vi "MaxiGauge EPICS.vi"() -> ()   [LabVIEW 2015]
uses:
  <vilib>/Platform/TimedLoop/XDataNode/timing_clust.ctl
  <vilib>/Platform/TimedLoop/XDataNode/nitl_modes.ctl
  <vilib>/Platform/TimedLoop/XDataNode/wakeup.ctl
  <userlib>/caLab/Private/Get_PV-1D.vi
  <userlib>/caLab/Private/Put_DBL-1D_PV-1D.vi
  <vilib>/platform/TimedLoop/XDataNode/XDataNode.xnode
  <vilib>/Platform/TimedLoop/XDataNode/XDNodeRunTimeDep.lvlib
panel:
  out "Finished Late? [i-1]":bool
  out "Actual Start [i]":i64
  out "Relay E":string
  out "Error out":errorcluster
  out "Maxigauge COMPORT":string
  out "APX:SEN6_STS":bool
  out "APX:SEN5_STS":bool
  out "APX:SEN4_STS":bool
  out "APX:SEN3_STS":bool
  out "APX:SEN2_STS":bool
  out "APX:SEN1_STS":bool
  out "APX:SEN6_VAL":dbl
  out "APX:SEN5_VAL":dbl
  out "APX:SEN4_VAL":dbl format="%#_3g"
  out "APX:SEN3_VAL":dbl format="%#_3g"
  out "APX:SEN2_VAL":dbl format="%#_3g"
  out "APX:SEN1_VAL":dbl
  out "APX:SEN6_OFF":bool
  out "APX:SEN6_ON":bool
  out "APX:SEN5_OFF":bool
  out "APX:SEN5_ON":bool
  out "APX:SEN4_OFF":bool
  out "APX:SEN4_ON":bool
  out "APX:SEN3_OFF":bool
  out "APX:SEN3_ON":bool
  out "APX:SEN2_OFF":bool
  out "APX:SEN2_ON":bool
  out "APX:SEN1_OFF":bool
  out "APX:SEN1_ON":bool
  out "APX:SP_SES100":bool
  out "MaxiGauge":dbl[](array[numeric])
  out "P torr":dbl[](array[numeric])
  in  "STOP":bool
  # "Ch 1\nGMP\nCh 6\nGMP\nCh 2\nGCC\nCh 4\nGHC\nCh 5\nGHC\n\nGMP"
  # "Send measured values to EPICS [COM8]"
  # "Relay E"
  # "K"
  # "EPICS PV name"
  # "N"
  # "APX:HPC100"
  # "APX:HPC100"
  # "APX:HPC01"
  # "APX:HPC"
  # "APX:HPC"
  # "N"
  # "APX:AP1"
  # "APX:PREP"
  # "APX:AP2"
  # "APX:Tsample"
  # "APX:AP1"
  # "APX:Tpiezo"
  # "APX:Thpc"
  # "APX:AP2"
  # "APX:PREP"
  # "APX:HPC01"
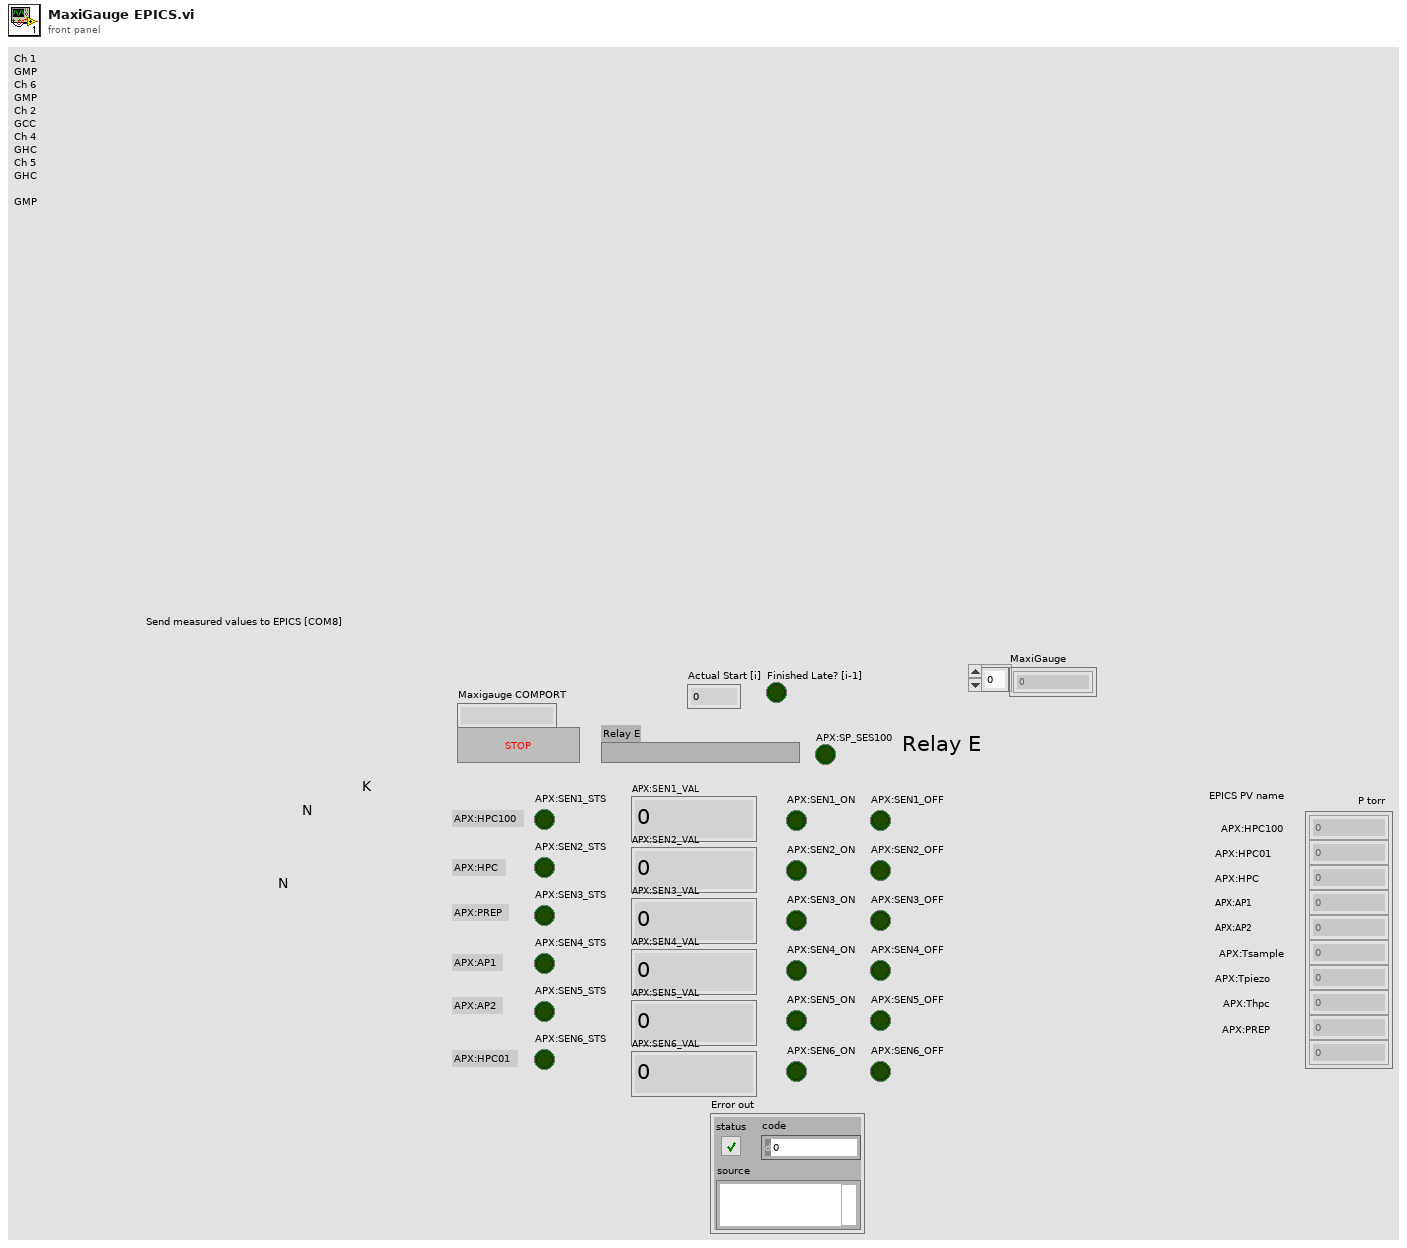
[diagram p1: front panel]
types:
  T1 = typedef "XDNodeRunTimeDep.lvlib/timing_clust.ctl" = cluster{"Expected End [f-1]":u64, "Actual End [f-1]":u64, "Finished Late? [f-1]":bool, "Expected End [i-1]":u64, "Actual End [i-1]":u64, "Finished Late? [i-1]":bool, "Expected Start [i]":u64, "Actual Start [i]":u64, "Expected Start [f]":u64, "Actual Start [f]":u64, "Source Name":string, "Structure Name":string, "Period":i64, "Deadline":i64, "Offset":i64, "Start":i64, "Priority":i32, "Timeout":i32, "Mode":T2, "Wakeup Reason":T3, "Error":errorcluster, "Source Type":string, "Secondary Source Type":string, "Global End Time":u64, "Global Start Time":u64, "Frame Duration":u64, "Iteration Duration":u64, "Assigned CPU":i32, "I/O Scan Engine Mode":u32}
  T2 = typedef "XDNodeRunTimeDep.lvlib/nitl_modes.ctl" = enum32{"No Change", "Process missed periods, maintain original phase", "Discard missed periods, maintain original phase", "Process missed periods, ignore original phase", "Discard missed periods, ignore original phase"}
  T3 = typedef "XDNodeRunTimeDep.lvlib/wakeup.ctl" = enum32{"Normal", "Aborted", "Asynchronous wakeup", "Timing source error", "Timed loop error", "Timeout"}
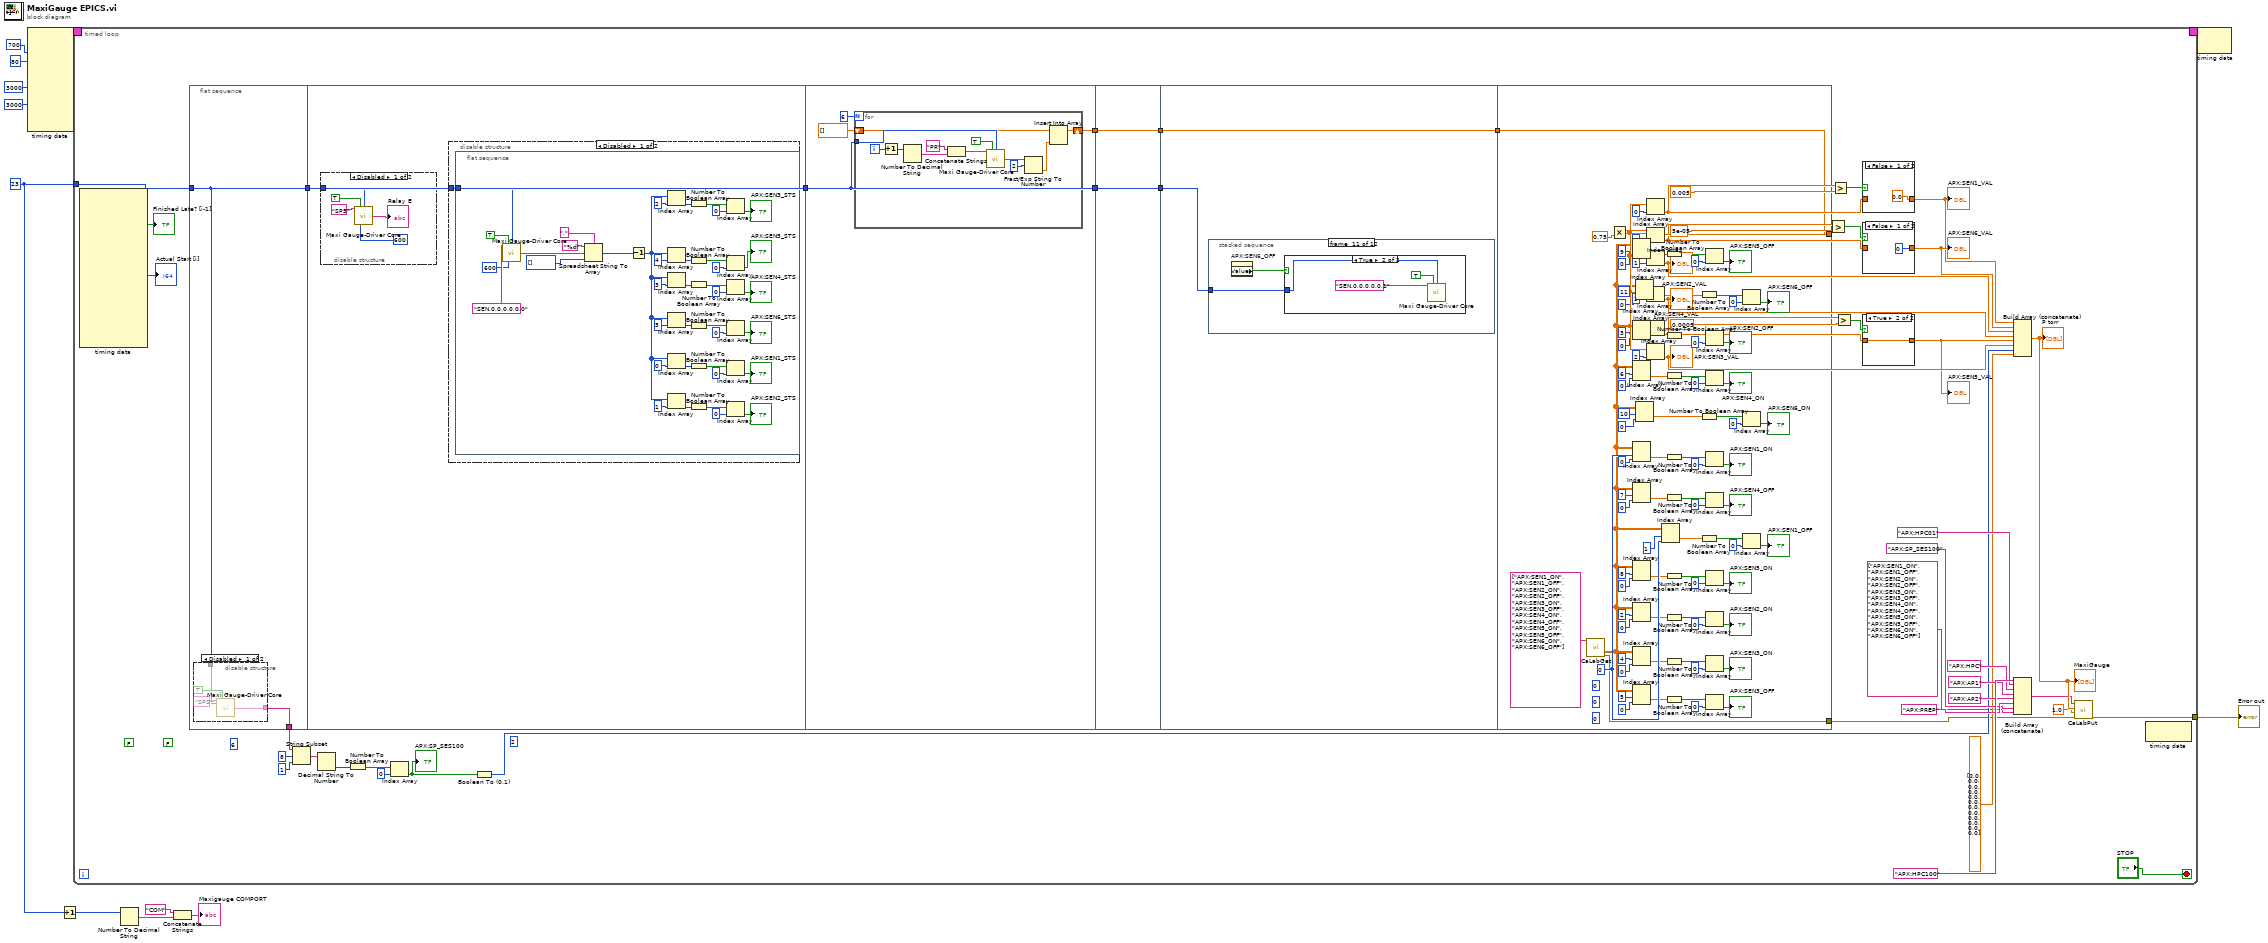
[diagram p0: block diagram]
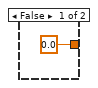
[diagram p2: hidden frame]
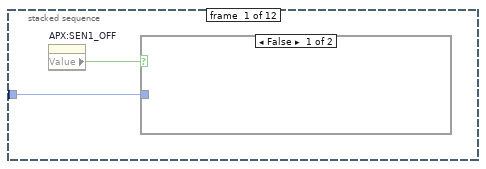
[diagram p6: hidden frame]
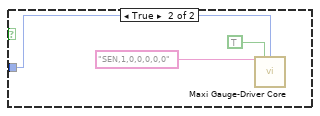
[diagram p7: hidden frame]
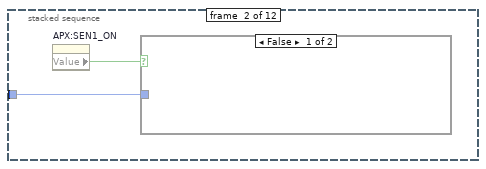
[diagram p8: hidden frame]
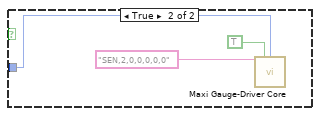
[diagram p9: hidden frame]
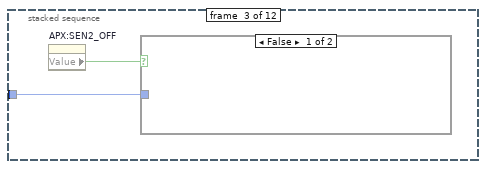
[diagram p10: hidden frame]
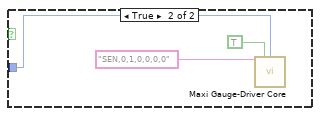
[diagram p11: hidden frame]
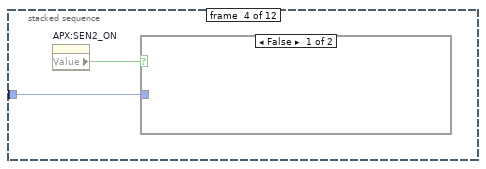
[diagram p12: hidden frame]
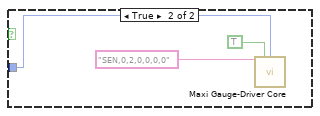
[diagram p13: hidden frame]
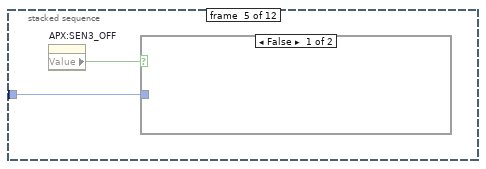
[diagram p14: hidden frame]
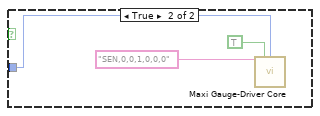
[diagram p15: hidden frame]
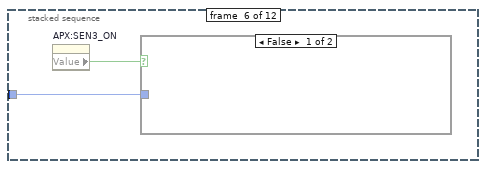
[diagram p16: hidden frame]
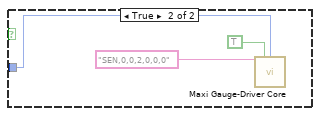
[diagram p17: hidden frame]
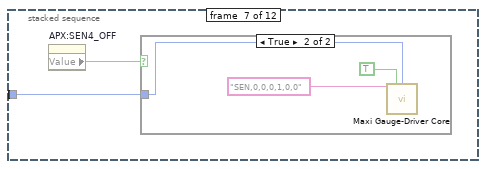
[diagram p18: hidden frame]
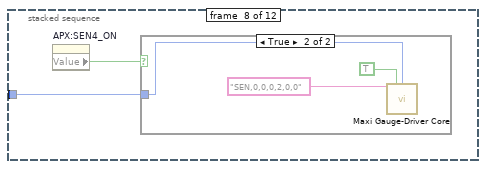
[diagram p20: hidden frame]
diagram:
  w8 = 23 ("Port")
  n1 = node-c288(i64 700 ("Period"), 80 ("Priority"), i64 3000 ("Deadline"), 3000 ("Timeout")) -> (w12:T1)  [unwired: 6 in]
  n2 = Increment(x=w8) -> (x+1=w7:i32)
  n3 = timed-loop {
    tunnel: w8 -> [w48]
    timing: w12 -> [_]
    timing-out: [_] -> w11
    tunnel: [w20] -> w3
    stop <- "STOP" stop-if-true
    (unwired) FALSE ("SES-100HVoff")
    (unwired) FALSE ("SES-100HVon")
    (unwired) 6
    (unwired) 2 ("index")
    n4 = node-c288() -> (→"Finished Late? [i-1]":bool, →"Actual Start [i]":i64)  [unwired: 1 in, 15 out]
    n5 = flat-sequence {
      tunnel: w48 -> [w73]
      tunnel: [w73] -> w15
      tunnel: [w74] -> w14
      tunnel: [w79] -> w47
      tunnel: w15 -> [w79]
      tunnel: w47 -> [w126]
      tunnel: [w127] -> w25
      tunnel: [w126] -> w24
      tunnel: w25 -> [w143]
      tunnel: [w143] -> w19
      tunnel: w24 -> [w142]
      tunnel: [w142] -> w17
      tunnel: w19 -> [w145]
      tunnel: [w145] -> w18
      tunnel: w17 -> [w144]
      tunnel: [w280] -> w60
      tunnel: w18 -> [w280]
      tunnel: [w206] -> w21
      frame #0 {
        n6 = disable-structure shown="Disabled" {
          disable-tunnel: [w76 _] -> w74
          disable-tunnel: w73 -> [w75 _]
          frame Disabled {
            n7 = call "Maxi Gauge-Driver Core.vi"("Command"="SPS", "Write/Read"=TRUE, "Port"=w75) -> ("String Out"=w76:string)  [unwired: 3 in, 9 out]
          }
          frame Enabled {
          }
        }
      }
      frame #1 {
        n8 = disable-structure shown="Disabled" {
          disable-tunnel: w79 -> [w124 _]
          frame Disabled {
            n9 = call "Maxi Gauge-Driver Core.vi"("Command"="SP5", "Write/Read"=TRUE, "Port"=w124, "Timeout [ms]"=u32 600) -> ("String Out"=→"Relay E":string)  [unwired: 2 in, 9 out]
          }
          frame Enabled {
          }
        }
        n10 = disable-structure shown="Disabled" {
          disable-tunnel: w79 -> [w80 _]
          frame Disabled {
            n11 = flat-sequence {
              tunnel: w80 -> [w82]
              frame #0 {
                n12 = call "Maxi Gauge-Driver Core.vi"("Command"="SEN,0,0,0,0,0,0", "Write/Read"=TRUE, "Port"=w82, "Timeout [ms]"=u32 600) -> ("String Out"=w117:string)  [unwired: 2 in, 9 out]
                n13 = Spreadsheet String To Array(delimiter (Tab)=",", format string="%d", spreadsheet string=w117, array type (2D Dbl)=i16[] []) -> (array=w113:i16[])
                n14 = Decrement(x=w113) -> (x-1=w88:i16[])
                n15 = Index Array(array=w88, index=2) -> (element=w103:i16)
                n16 = Index Array(array=w88, index=4) -> (element=w95:i16)
                n17 = Index Array(array=w88, index=3) -> (element=w99:i16)
                n18 = Index Array(array=w88, index=5) -> (element=w91:i16)
                n19 = Index Array(array=w88, index=0) -> (element=w112:i16)
                n20 = Index Array(array=w88, index=1) -> (element=w107:i16)
                n21 = Number To Boolean Array(number=w103) -> (Boolean array=w102:bool[])
                n22 = Number To Boolean Array(number=w95) -> (Boolean array=w94:bool[])
                n23 = Number To Boolean Array(number=w99) -> (Boolean array=w98:bool[])
                n24 = Number To Boolean Array(number=w91) -> (Boolean array=w90:bool[])
                n25 = Number To Boolean Array(number=w112) -> (Boolean array=w111:bool[])
                n26 = Number To Boolean Array(number=w107) -> (Boolean array=w106:bool[])
                n27 = Index Array(array=w102, index=0) -> (element=→"APX:SEN3_STS":bool)
                n28 = Index Array(array=w94, index=0) -> (element=→"APX:SEN5_STS":bool)
                n29 = Index Array(array=w98, index=0) -> (element=→"APX:SEN4_STS":bool)
                n30 = Index Array(array=w90, index=0) -> (element=→"APX:SEN6_STS":bool)
                n31 = Index Array(array=w111, index=0) -> (element=→"APX:SEN1_STS":bool)
                n32 = Index Array(array=w106, index=0) -> (element=→"APX:SEN2_STS":bool)
              }
            }
          }
          frame Enabled {
          }
        }
      }
      frame #2 {
        n33 = for {
          N: 6 -> [_]
          tunnel: w126 -> [w133]
          shift-right: [w130] -> w127
          shift-left: dbl[] [] -> [w131]
          i -> [w135]
          n34 = Increment(x=w135) -> (x+1=w138:i32)
          n35 = Number To Decimal String(number=w138) -> (decimal integer string=w141:string)  [unwired: 1 out]
          n36 = Concatenate Strings("PR", w141) -> (w139:string)
          n37 = call "Maxi Gauge-Driver Core.vi"("Command"=w139, "Write/Read"=TRUE, "Port"=w133) -> ("String Out"=w137:string)  [unwired: 3 in, 9 out]
          n38 = Fract/Exp String To Number(string=w137, offset=2 ("offset (0)")) -> (number=w132:dbl)  [unwired: 3 out]
          n39 = Insert Into Array(array=w131, new element=w132) -> (w130:dbl[])  [unwired: 1 in]
        }
      }
      frame #3 {
      }
      frame #4 {
        n40 = stacked-sequence {
          tunnel: w144 -> [w146 w151 w156 w161 w166 w171 w176 w181 w186 w191 w196 w201]
          frame #0 {
            n41 = property on="APX:SEN1_OFF" class="Bool (strict)"() -> ("Value"=w147:bool)  [unwired: 2 in, 2 out]
            n42 = case shown="False" w147 {
              tunnel: w146 -> [_ w148]
              frame False {
              }
              frame True {
                n43 = call "Maxi Gauge-Driver Core.vi"("Command"="SEN,1,0,0,0,0,0", "Write/Read"=TRUE, "Port"=w148) -> ()  [unwired: 3 in, 10 out]
              }
            }
          }
          frame #1 {
            n44 = property on="APX:SEN1_ON" class="Bool (strict)"() -> ("Value"=w152:bool)  [unwired: 2 in, 2 out]
            n45 = case shown="False" w152 {
              tunnel: w151 -> [_ w153]
              frame False {
              }
              frame True {
                n46 = call "Maxi Gauge-Driver Core.vi"("Command"="SEN,2,0,0,0,0,0", "Write/Read"=TRUE, "Port"=w153) -> ()  [unwired: 3 in, 10 out]
              }
            }
          }
          frame #2 {
            n47 = property on="APX:SEN2_OFF" class="Bool (strict)"() -> ("Value"=w157:bool)  [unwired: 2 in, 2 out]
            n48 = case shown="False" w157 {
              tunnel: w156 -> [_ w159]
              frame False {
              }
              frame True {
                n49 = call "Maxi Gauge-Driver Core.vi"("Command"="SEN,0,1,0,0,0,0", "Write/Read"=TRUE, "Port"=w159) -> ()  [unwired: 3 in, 10 out]
              }
            }
          }
          frame #3 {
            n50 = property on="APX:SEN2_ON" class="Bool (strict)"() -> ("Value"=w162:bool)  [unwired: 2 in, 2 out]
            n51 = case shown="False" w162 {
              tunnel: w161 -> [_ w164]
              frame False {
              }
              frame True {
                n52 = call "Maxi Gauge-Driver Core.vi"("Command"="SEN,0,2,0,0,0,0", "Write/Read"=TRUE, "Port"=w164) -> ()  [unwired: 3 in, 10 out]
              }
            }
          }
          frame #4 {
            n53 = property on="APX:SEN3_OFF" class="Bool (strict)"() -> ("Value"=w167:bool)  [unwired: 2 in, 2 out]
            n54 = case shown="False" w167 {
              tunnel: w166 -> [_ w168]
              frame False {
              }
              frame True {
                n55 = call "Maxi Gauge-Driver Core.vi"("Command"="SEN,0,0,1,0,0,0", "Write/Read"=TRUE, "Port"=w168) -> ()  [unwired: 3 in, 10 out]
              }
            }
          }
          frame #5 {
            n56 = property on="APX:SEN3_ON" class="Bool (strict)"() -> ("Value"=w172:bool)  [unwired: 2 in, 2 out]
            n57 = case shown="False" w172 {
              tunnel: w171 -> [_ w174]
              frame False {
              }
              frame True {
                n58 = call "Maxi Gauge-Driver Core.vi"("Command"="SEN,0,0,2,0,0,0", "Write/Read"=TRUE, "Port"=w174) -> ()  [unwired: 3 in, 10 out]
              }
            }
          }
          frame #6 {
            n59 = property on="APX:SEN4_OFF" class="Bool (strict)"() -> ("Value"=w177:bool)  [unwired: 2 in, 2 out]
            n60 = case shown="True" w177 {
              tunnel: w176 -> [_ w179]
              frame False {
              }
              frame True {
                n61 = call "Maxi Gauge-Driver Core.vi"("Command"="SEN,0,0,0,1,0,0", "Write/Read"=TRUE, "Port"=w179) -> ()  [unwired: 3 in, 10 out]
              }
            }
          }
          frame #7 {
            n62 = property on="APX:SEN4_ON" class="Bool (strict)"() -> ("Value"=w182:bool)  [unwired: 2 in, 2 out]
            n63 = case shown="True" w182 {
              tunnel: w181 -> [_ w184]
              frame False {
              }
              frame True {
                n64 = call "Maxi Gauge-Driver Core.vi"("Command"="SEN,0,0,0,2,0,0", "Write/Read"=TRUE, "Port"=w184) -> ()  [unwired: 3 in, 10 out]
              }
            }
          }
          frame #8 {
            n65 = property on="APX:SEN5_OFF" class="Bool (strict)"() -> ("Value"=w187:bool)  [unwired: 2 in, 2 out]
            n66 = case shown="True" w187 {
              tunnel: w186 -> [_ w189]
              frame False {
              }
              frame True {
                n67 = call "Maxi Gauge-Driver Core.vi"("Command"="SEN,0,0,0,0,1,0", "Write/Read"=TRUE, "Port"=w189) -> ()  [unwired: 3 in, 10 out]
              }
            }
          }
          frame #9 {
            n68 = property on="APX:SEN5_ON" class="Bool (strict)"() -> ("Value"=w192:bool)  [unwired: 2 in, 2 out]
            n69 = case shown="True" w192 {
              tunnel: w191 -> [_ w194]
              frame False {
              }
              frame True {
                n70 = call "Maxi Gauge-Driver Core.vi"("Command"="SEN,0,0,0,0,2,0", "Write/Read"=TRUE, "Port"=w194) -> ()  [unwired: 3 in, 10 out]
              }
            }
          }
          frame #10 {
            n71 = property on="APX:SEN6_OFF" class="Bool (strict)"() -> ("Value"=w197:bool)  [unwired: 2 in, 2 out]
            n72 = case shown="True" w197 {
              tunnel: w196 -> [_ w199]
              frame False {
              }
              frame True {
                n73 = call "Maxi Gauge-Driver Core.vi"("Command"="SEN,0,0,0,0,0,1", "Write/Read"=TRUE, "Port"=w199) -> ()  [unwired: 3 in, 10 out]
              }
            }
          }
          frame #11 {
            n74 = property on="APX:SEN6_ON" class="Bool (strict)"() -> ("Value"=w202:bool)  [unwired: 2 in, 2 out]
            n75 = case shown="True" w202 {
              tunnel: w201 -> [_ w204]
              frame False {
              }
              frame True {
                n76 = call "Maxi Gauge-Driver Core.vi"("Command"="SEN,0,0,0,0,0,2", "Write/Read"=TRUE, "Port"=w204) -> ()  [unwired: 3 in, 10 out]
              }
            }
          }
        }
      }
      frame #5 {
        (unwired) 0 ("index (col)")
        w269 = 0 ("index")
        (unwired) 0 ("disabled index (col)")
        (unwired) 0 ("index (row)")
        n77 = call-poly "CaLabGet.vi"("PV Names"=string[] ["APX:SEN1_ON", "APX:SEN1_OFF", "APX:SEN2_ON", "APX:SEN2_OFF", "APX:SEN3_ON", "APX:SEN3_OFF", "APX:SEN4_ON", "APX:SEN4_OFF", "APX:SEN5_ON", "APX:SEN5_OFF", "APX:SEN6_ON", "APX:SEN6_OFF"]) -> ("Value Array (number)"=w228:dbl[][], "Error out"=w206:errorcluster)  [unwired: 8 in, 5 out]
        n78 = Index Array(array=w228, index (row)=9 ("disabled index (col)"), index (col)=0) -> (element=w211:dbl)
        n79 = Index Array(array=w228, index (row)=3 ("disabled index (col)"), index (col)=0) -> (element=w223:dbl)
        n80 = Index Array(array=w228, index (row)=6 ("disabled index (col)"), index (col)=0) -> (element=w217:dbl)
        n81 = Index Array(array=w228, index (row)=w269, index (col)=0 ("disabled index (col)")) -> (element=w277:dbl)
        n82 = Index Array(array=w228, index (row)=7 ("disabled index (col)"), index (col)=0) -> (element=w215:dbl)
        n83 = Index Array(array=w228, index (row)=8 ("disabled index (col)"), index (col)=0) -> (element=w213:dbl)
        n84 = Index Array(array=w228, index (row)=2 ("disabled index (col)"), index (col)=0) -> (element=w225:dbl)
        n85 = Index Array(array=w228, index (row)=4 ("disabled index (col)"), index (col)=0) -> (element=w221:dbl)
        n86 = Index Array(array=w228, index (row)=5 ("disabled index (col)"), index (col)=0) -> (element=w219:dbl)
        n87 = Index Array(array=w228, index (row)=11 ("disabled index (col)"), index (col)=0) -> (element=w207:dbl)
        n88 = Index Array(array=w228, index (row)=10 ("disabled index (col)"), index (col)=0) -> (element=w209:dbl)
        n89 = Index Array(array=w228, index (row)=1 ("disabled index (col)"), index (col)=w269) -> (element=w273:dbl)
        n90 = Number To Boolean Array(number=w211) -> (Boolean array=w239:bool[])
        n91 = Number To Boolean Array(number=w223) -> (Boolean array=w263:bool[])
        n92 = Number To Boolean Array(number=w217) -> (Boolean array=w251:bool[])
        n93 = Number To Boolean Array(number=w277) -> (Boolean array=w276:bool[])
        n94 = Number To Boolean Array(number=w215) -> (Boolean array=w247:bool[])
        n95 = Number To Boolean Array(number=w213) -> (Boolean array=w243:bool[])
        n96 = Number To Boolean Array(number=w225) -> (Boolean array=w267:bool[])
        n97 = Number To Boolean Array(number=w221) -> (Boolean array=w259:bool[])
        n98 = Number To Boolean Array(number=w219) -> (Boolean array=w255:bool[])
        n99 = Number To Boolean Array(number=w207) -> (Boolean array=w231:bool[])
        n100 = Number To Boolean Array(number=w209) -> (Boolean array=w235:bool[])
        n101 = Number To Boolean Array(number=w273) -> (Boolean array=w272:bool[])
        n102 = Index Array(array=w239, index=0) -> (element=→"APX:SEN5_OFF":bool)
        n103 = Index Array(array=w263, index=0) -> (element=→"APX:SEN2_OFF":bool)
        n104 = Index Array(array=w251, index=0) -> (element=→"APX:SEN4_ON":bool)
        n105 = Index Array(array=w276, index=0) -> (element=→"APX:SEN1_ON":bool)
        n106 = Index Array(array=w247, index=0) -> (element=→"APX:SEN4_OFF":bool)
        n107 = Index Array(array=w243, index=0) -> (element=→"APX:SEN5_ON":bool)
        n108 = Index Array(array=w267, index=0) -> (element=→"APX:SEN2_ON":bool)
        n109 = Index Array(array=w259, index=0) -> (element=→"APX:SEN3_ON":bool)
        n110 = Index Array(array=w255, index=0) -> (element=→"APX:SEN3_OFF":bool)
        n111 = Index Array(array=w231, index=0) -> (element=→"APX:SEN6_OFF":bool)
        n112 = Index Array(array=w235, index=0) -> (element=→"APX:SEN6_ON":bool)
        n113 = Index Array(array=w272, index=0) -> (element=→"APX:SEN1_OFF":bool)
      }
    }
    n114 = String Subset(string=w14, offset (0)=8, length (rest)=1 ("length (rest)")) -> (substring=w41:string)
    n115 = Decimal String To Number(string=w41) -> (number=w42:i32)  [unwired: 2 in, 1 out]
    n116 = Number To Boolean Array(number=w42) -> (Boolean array=w44:bool[])
    n117 = Index Array(array=w44, index=0) -> (element=w40:bool)
    "APX:SP_SES100" <- w40
    n118 = Boolean To (0,1)(Boolean=w40) -> (0, 1=w31:i16)
    n119 = Multiply(x=w60, y=0.75) -> (x*y=w50:dbl[])
    n120 = Index Array(array=w50, index=0) -> (element=w39:dbl)
    n121 = Index Array(array=w50, index=5) -> (element=w36:dbl)
    n122 = Index Array(array=w50, index=1) -> (element=w38:dbl)
    "APX:SEN2_VAL" <- w38
    n123 = Index Array(array=w50, index=3) -> (element=w37:dbl)
    "APX:SEN4_VAL" <- w37
    n124 = Index Array(array=w50, index=4) -> (element=w29:dbl)
    n125 = Index Array(array=w50, index=2) -> (element=w33:dbl)
    "APX:SEN3_VAL" <- w33
    n126 = Greater?(x=w36, y=5e-05) -> (0:w64:bool)
    n127 = Greater?(x=w39, y=0.005) -> (0:w61:bool)
    n128 = Greater?(x=w29, y=0.0005) -> (0:w30:bool)
    n129 = case shown="False" w61 {
      tunnel: [0.0 w282] -> w26
      tunnel: w39 -> [_ w282]
      frame False {
      }
      frame True {
      }
    }
    "APX:SEN1_VAL" <- w26
    n130 = case shown="False" w64 {
      tunnel: [0 w284] -> w27
      tunnel: w36 -> [_ w284]
      frame False {
      }
      frame True {
      }
    }
    "APX:SEN6_VAL" <- w27
    n131 = case shown="True" w30 {
      tunnel: [0.0 w72] -> w28
      tunnel: w29 -> [_ w72]
      frame False {
      }
      frame True {
      }
    }
    "APX:SEN5_VAL" <- w28
    n132 = Build Array (concatenate)("APX:HPC100", "APX:HPC01", "APX:HPC", "APX:AP1", "APX:AP2", "APX:PREP", "APX:SP_SES100" ("element"), string[] ["APX:SEN1_ON", "APX:SEN1_OFF", "APX:SEN2_ON", "APX:SEN2_OFF", "APX:SEN3_ON", "APX:SEN3_OFF", "APX:SEN4_ON", "APX:SEN4_OFF", "APX:SEN5_ON", "APX:SEN5_OFF", "APX:SEN6_ON", "APX:SEN6_OFF"]) -> (w57:string[])
    n133 = Build Array (concatenate)(w26, w27, w38, w37, w28, w33, w31, dbl[] [0.0, 0.0, 0.0, 0.0, 0.0, 0.0, 0.0, 0.0, 0.0, 0.0, 0.0, 0.0]) -> (w58:dbl[])
    "P torr" <- w58
    "MaxiGauge" <- w58
    n134 = call-poly <userlib>:"CaLabPut.vi"("Error in (no error)"=w21, "Timeout (3)"=1.0, "Values"=w58, "PV Names"=w57) -> ("Error out"=w20:errorcluster)  [unwired: 4 in, 3 out]
    n135 = node-c288() -> ()  [unwired: 1 in, 1 out]
  }
  "Error out" <- w3
  n136 = Number To Decimal String(number=w7) -> (decimal integer string=w6:string)  [unwired: 1 in]
  n137 = Concatenate Strings("COM" ("string"), w6) -> (→"Maxigauge COMPORT":string)
  n138 = node-c288(w11) -> ()  [unwired: 1 out]
